vi "Read Individual Limit Test Result.vi"(8 "error in (no error)":errorcluster, 9 "Limit Test Number (1)":i32=1, 10 "Channel (0: Channel 1)":i32(ring) items=["Channel 1", "Channel 2"], 11 "VISA resource name":refnum<visa-resource-name>) -> (0 "error out":errorcluster, 2 "Limit Test Failed?":bool, 3 "VISA resource name out":refnum<visa-resource-name>)   [LabVIEW 2023, in "Agilent B2900 Series.lvlib"]
doc: "Read the result of specified Limit Test.\n\n<B>Note:</B> \n(1) Use this VI only with other low-level VIs. The high-level VIs automatically incorporate this functionality. This VI does not check the instrument status. \n(2) This VI is not applicable for Agilent models B2961A, B2962A, B2961B, B2962B, B2961C and B2962C."
uses:
  Agilent B2900 Series.lvlib
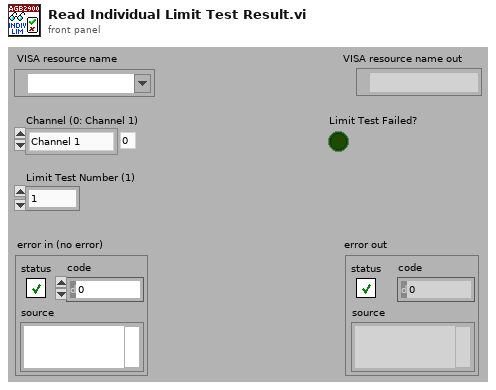
[diagram p1: front panel]
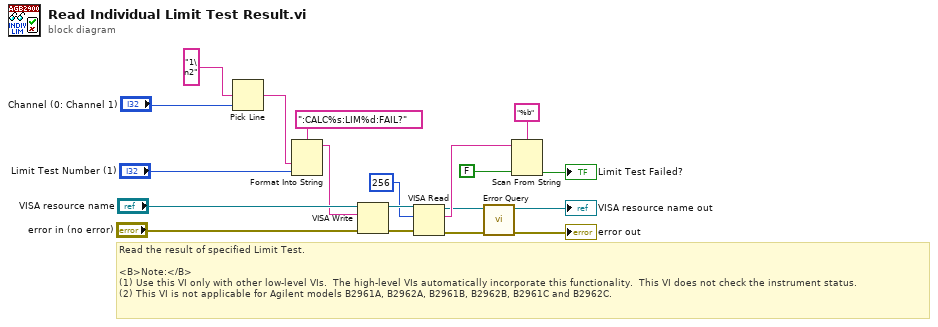
[diagram p0: block diagram]
diagram:
  # "Read the result of specified Limit Test.\n\n<B>Note:</B> \n(1) Use this VI only with other low-level VIs.  The high-level VIs automatically incorporate this functionality.  This VI does not check the instrument status.   \n(2) This VI is not applicable for Agilent models B2961A, B2962A, B2961B, B2962B, B2961C and B2962C."
  n1 = Pick Line(multi-line string="1\n2" ("string (\"\")"), line index="Channel (0: Channel 1)") -> (output string=w16:string)  [unwired: 1 in]
  n2 = Format Into String(format string=":CALC%s:LIM%d:FAIL?", w16, "Limit Test Number (1)") -> (resulting string=w12:string)  [unwired: 2 in, 1 out]
  n3 = VISA Write(VISA resource name="VISA resource name", write buffer=w12, error in (no error)="error in (no error)") -> (VISA resource name out=w11:refnum<visa-resource-name>, error out=w10:errorcluster)  [unwired: 1 out]
  n4 = VISA Read(VISA resource name=w11, byte count=u32 256, error in (no error)=w10) -> (VISA resource name out=w1:refnum<visa-resource-name>, read buffer=w9:string, error out=w2:errorcluster)  [unwired: 1 out]
  n5 = call "Error Query.vi"("error in (no error)"=w2, "VISA resource name"=w1) -> ("error out"=→"error out":errorcluster, "VISA resource name out"=→"VISA resource name out":refnum<visa-resource-name>)  [unwired: 6 in, 2 out]
  n6 = Scan From String(format string="%b", input string=w9, default 1=FALSE ("default value 1")) -> (output 1=→"Limit Test Failed?":bool)  [unwired: 2 in, 3 out]
